vi "Spark test.vi"() -> ()   [LabVIEW 2018]
uses:
  <vilib>/DAQmx/write.llb/DAQmx Write (Digital Bool 1Line 1Point).vi
  <vilib>/DAQmx/create/channels.llb/DAQmx Create Channel (DO-Digital Output).vi
  <vilib>/DAQmx/miscellaneous.llb/DAQmx Fill In Error Info.vi
panel:
  in  "Stop Button":bool
  in  "Spark":bool
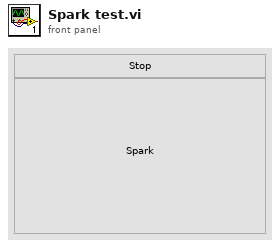
[diagram p1: front panel]
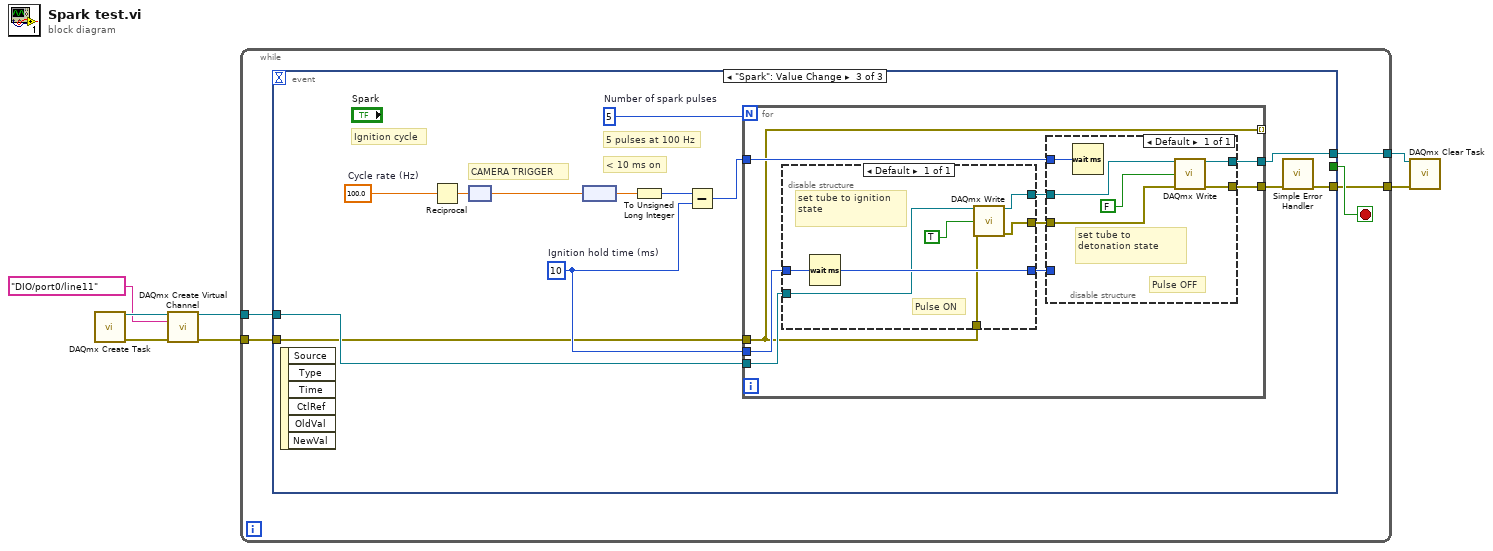
[diagram p0: block diagram]
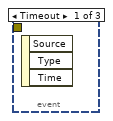
[diagram p2: hidden frame]
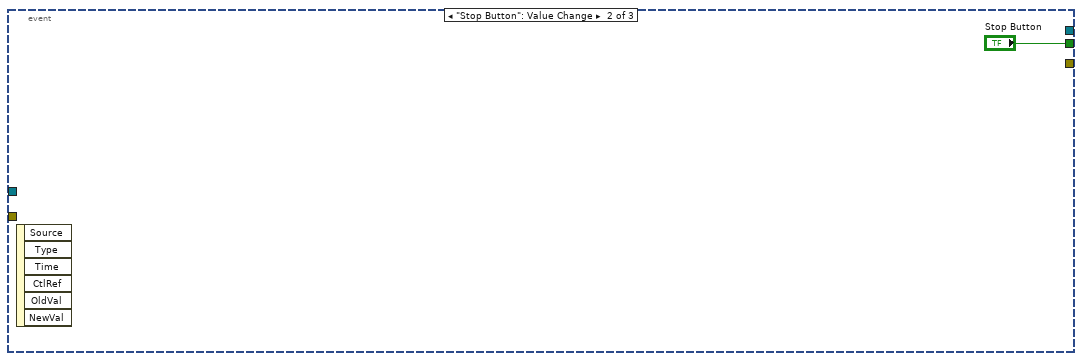
[diagram p3: hidden frame]
diagram:
  n1 = call <vilib>:"DAQmx Create Task.vi"() -> ("task out"=w7:refnum<k21>, "error out"=w6:errorcluster)  [unwired: 14 in]
  n2 = call-poly <vilib>:"DAQmx Create Virtual Channel.vi"("task in"=w7, "lines"=tag "DIO/port0/line11", "error in"=w6) -> ("task out"=w4:refnum<k21>, "error out"=w3:errorcluster)  [unwired: 11 in]
  n3 = while {
    tunnel: w4 -> [w11]
    tunnel: w3 -> [w10]
    tunnel: [w9] -> w2
    tunnel: [w8] -> w1
    stop <- w12 stop-if-true
    n4 = event shown="[2] \"Spark\": Value Change" {
      selector: _ -> [_ _ _]
      dyn-events: _ -> [_ _ _]
      timeout: _ -> [_ _ _]
      tunnel: [_ "Stop Button" _] -> w12
      tunnel: w11 -> [_ _ w18]
      tunnel: w10 -> [_ _ w17]
      tunnel: [_ _ w15] -> w9
      tunnel: [_ _ w14] -> w8
      event Timeout {
        n5 = event-data() -> ()  [unwired: 1 in, 3 out]
      }
      event "Stop Button": Value Change {
        n6 = event-data() -> ()  [unwired: 1 in, 6 out]
      }
      event "Spark": Value Change {
        w25 = u32 10  # Ignition hold time (ms)
        w20 = 100.0  # Cycle rate (Hz)
        w19 = 5  # Number of spark pulses
        # "CAMERA TRIGGER"
        # "Ignition cycle"
        # "5 pulses at 100 Hz"
        # "< 10 ms on"
        n7 = event-data() -> ()  [unwired: 1 in, 6 out]
        n8 = Reciprocal(x=w20) -> (1/x=w21:dbl)
        n9 = node(w21) -> (w22:dbl[unit])
        n10 = node(w22) -> (w23:dbl)
        n11 = To Unsigned Long Integer(number=w23) -> (unsigned 32bit integer=w24:u32)
        n12 = Subtract(x=w24, y=w25) -> (x-y=w26:u32)
        n13 = for {
          N: w19 -> [_]
          tunnel: w25 -> [w35]
          tunnel: w26 -> [w34]
          tunnel: w18 -> [w28]
          tunnel: [w27] -> _ mode=indexing
          tunnel: [w30] -> w16
          tunnel: [w29] -> w15
          tunnel: w17 -> [w27]
          n14 = disable-structure shown="Default" {
            disable-tunnel: w35 -> [w48]
            disable-tunnel: [w47] -> w33
            disable-tunnel: [w45] -> w32
            disable-tunnel: [w44] -> w31
            disable-tunnel: w28 -> [w43]
            disable-tunnel: w27 -> [w42]
            frame Enabled {
              # "Pulse ON"
              # "set tube to ignition state"
              n15 = Wait (ms)(milliseconds to wait=w48) -> (millisecond timer value=w47:u32)
              n16 = call-poly <vilib>:"DAQmx Write.vi"("task/channels in"=w43, "data"=TRUE, "error in"=w42) -> ("task out"=w45:refnum<k21>, "error out"=w44:errorcluster)  [unwired: 10 in, 1 out]
            }
          }
          n17 = disable-structure shown="Default" {
            disable-tunnel: w34 -> [w41]
            disable-tunnel: w33 -> [_]
            disable-tunnel: w32 -> [w39]
            disable-tunnel: w31 -> [w38]
            disable-tunnel: [w37] -> w30
            disable-tunnel: [w36] -> w29
            frame Enabled {
              # "Pulse OFF"
              # "set tube to detonation state"
              n18 = Wait (ms)(milliseconds to wait=w41) -> ()  [unwired: 1 out]
              n19 = call-poly <vilib>:"DAQmx Write.vi"("task/channels in"=w39, "data"=FALSE, "error in"=w38) -> ("task out"=w36:refnum<k21>, "error out"=w37:errorcluster)  [unwired: 10 in, 1 out]
            }
          }
        }
        n20 = call <vilib>:"Simple Error Handler.vi"("error in (no error)"=w16) -> ("error out"=w14:errorcluster)  [unwired: 4 in, 4 out]
      }
    }
  }
  n21 = call <vilib>:"DAQmx Clear Task.vi"("task in"=w2, "error in"=w1) -> ()  [unwired: 13 in, 1 out]
